vi "niRFUtil FWK Configure Acquisition Timing_deprecated.vi"(3 "Measurement Delay, sec (0)":dbl format="%^.2e", 4 "Desired Delay, sec (0)":dbl format="%^.2e", 5 "Desired Time, sec":dbl=0.001 format="%^.2e") -> (0 "Post-Trigger Delay, sec":dbl format="%^.2e", 1 "Pre-Trigger Delay, sec":dbl format="%^.2e", 2 "Time, sec":dbl format="%^.2e")   [LabVIEW 2015, in "niRFUtil.lvlib"]
doc: "(c) Copyright 2006, National Instruments, Inc. This VI may not be duplicated, sold, or distributed without written consent from National Instruments."
uses:
  niRFUtil.lvlib
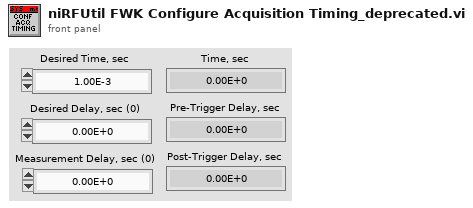
[diagram p1: front panel]
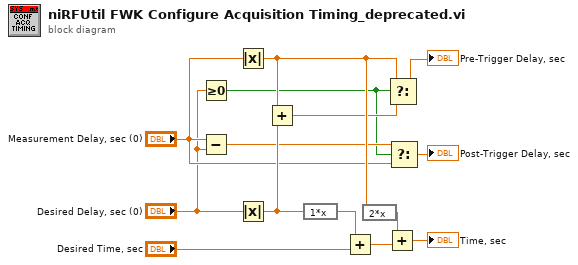
[diagram p0: block diagram]
diagram:
  n1 = Greater Or Equal To 0?(x="Desired Delay, sec (0)") -> (x >= 0?=w7:bool)
  n2 = Subtract(x="Measurement Delay, sec (0)", y="Desired Delay, sec (0)") -> (x-y=w8:dbl)
  n3 = Absolute Value(x="Measurement Delay, sec (0)") -> (abs(x)=w11:dbl)
  n4 = Absolute Value(x="Desired Delay, sec (0)") -> (abs(x)=w10:dbl)
  n5 = Add(x=w11, y=w10) -> (x+y=w9:dbl)
  n6 = expression code="1*x"(w10) -> (w12:dbl)
  n7 = Add(x=w12, y="Desired Time, sec") -> (x+y=w14:dbl)
  n8 = expression code="2*x"(w11) -> (w13:dbl)
  n9 = Add(x=w13, y=w14) -> (x+y=→"Time, sec":dbl)
  n10 = Select(t=w11, s=w7, f=w9) -> (s? t:f=→"Pre-Trigger Delay, sec":dbl)
  n11 = Select(t=w8, s=w7, f="Measurement Delay, sec (0)") -> (s? t:f=→"Post-Trigger Delay, sec":dbl)
